vi "3667_Can_4Motor.vi"(0 "Device Number(Rl)":u8, 1 "Control Mode":T1, 2 "Rear Left Motor Inverted":bool, 3 "Rear Right Motor Inverted":bool, 5 "Device Number(Rr)":u8, 7 "Device Number(Fl)":u8, 9 "Device Number(Fr)":u8, 11 "error in (no error)":errorcluster, 13 "Front Left Motor Inverted":bool, 14 "Front Right Motor Inverted":bool) -> (4 "RobotDriveDevRef":T2={"DevStatus"={"status"=FALSE, "code"=0, "source"=""}, "Motors[]"=[], "Square Inputs"=FALSE, "Max Output"=1.0}, 15 "error out":errorcluster)   [LabVIEW 2016]
uses:
  <vilib>/Rock Robotics/WPI/RobotDrive/WPI_RobotDriveDevRef.ctl
  <vilib>/Rock Robotics/WPI/MotorControl/WPI_MotorControlDeviceRef.ctl
  <vilib>/Rock Robotics/WPI/MotorControl/WPI_MotorControlType.ctl
  <vilib>/Rock Robotics/SystemInterfaces/DIO/FPGA_DIOPWMChannel.ctl
  <vilib>/Rock Robotics/WPI/PWM/WPI_PWMDeadband.ctl
  <vilib>/Rock Robotics/WPI/ThirdParty/CanMotor/TalonSRX/WPI_CANTalonSRX_APIControlMode.ctl
  <vilib>/Rock Robotics/WPI/SafetyOutput/WPI_SafetyOutputConfigMenu.ctl
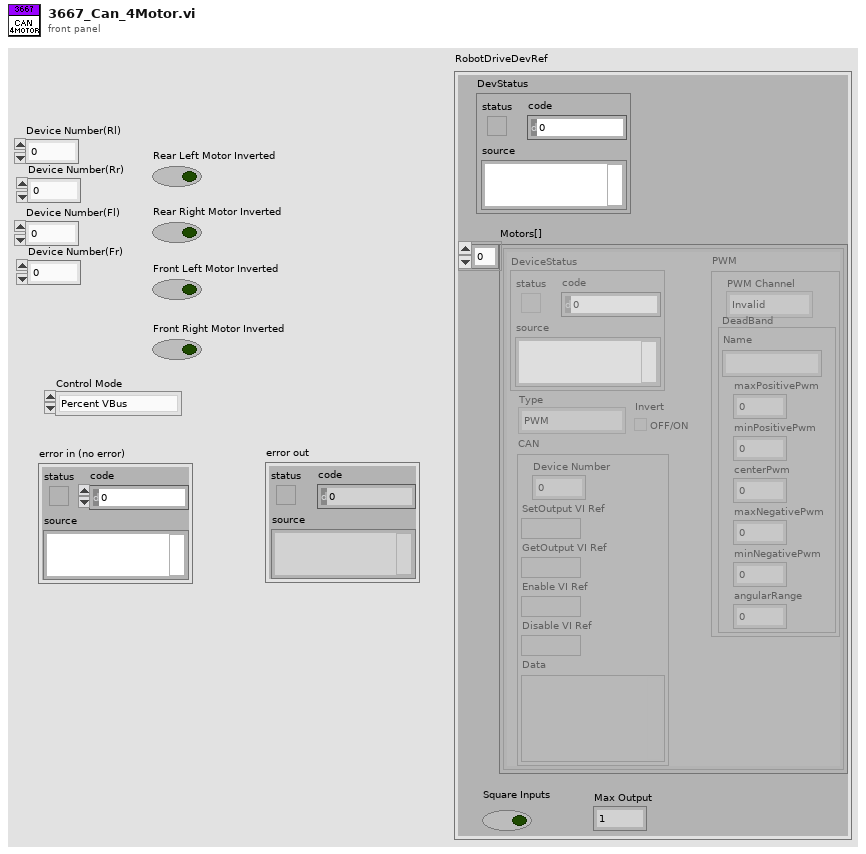
[diagram p1: front panel]
types:
  T1 = typedef "WPI_CANTalonSRX_APIControlMode.ctl" = enum8{"Percent VBus", "Speed", "Position", "Slave", "Unchanged / Invalid", "Voltage Compensation", "Current", "Motion Profile", "Motion Magic"}
  T2 = typedef "WPI_RobotDriveDevRef.ctl" = cluster{"DevStatus":errorcluster, "Motors[]":T3[], "Square Inputs":bool, "Max Output":dbl}
  T3 = typedef "WPI_MotorControlDeviceRef.ctl" = cluster{"DeviceStatus":errorcluster, "Type":T4, "PWM":cluster{"PWM Channel":T5, "DeadBand":T6}, "CAN":cluster{"Device Number":u8, "SetOutput VI Ref":variant, "GetOutput VI Ref":variant, "Enable VI Ref":variant, "Disable VI Ref":variant, "Data":variant}, "Invert":bool}
  T4 = typedef "WPI_MotorControlType.ctl" = enum16{"PWM", "CAN"}
  T5 = typedef "FPGA_DIOPWMChannel.ctl" = enum8{"PWM 0", "PWM 1", "PWM 2", "PWM 3", "PWM 4", "PWM 5", "PWM 6", "PWM 7", "PWM 8", "PWM 9", "PWM MXP 0", "PWM MXP 1", "PWM MXP 2", "PWM MXP 3", "PWM MXP 4", "PWM MXP 5", "PWM MXP 6", "PWM MXP 7", "PWM MXP 8", "PWM MXP 9", "Invalid"}
  T6 = typedef "WPI_PWMDeadband.ctl" = cluster{"Name":string, "maxPositivePwm":i32, "minPositivePwm":i32, "centerPwm":i32, "maxNegativePwm":i32, "minNegativePwm":i32, "angularRange":u16}
  T7 = typedef "WPI_SafetyOutputConfigMenu.ctl" = enum16{"Enable", "Disable"}
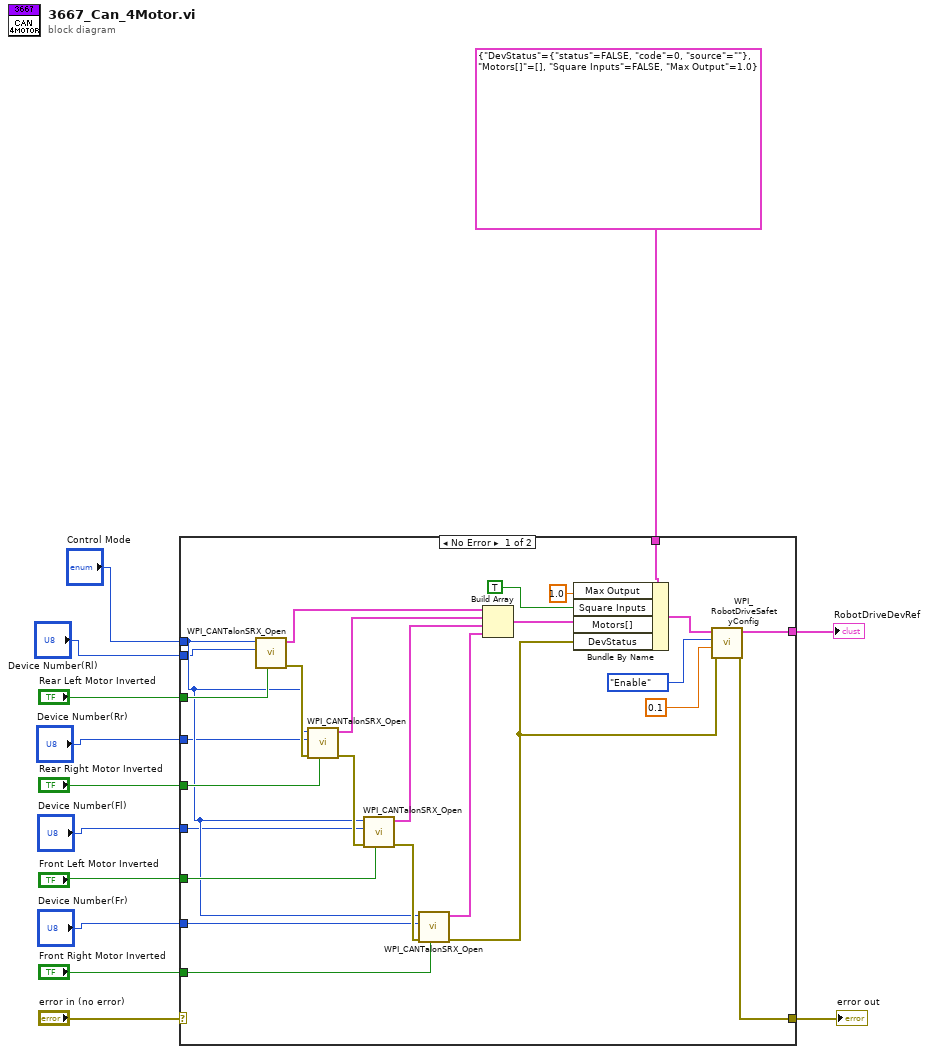
[diagram p0: block diagram]
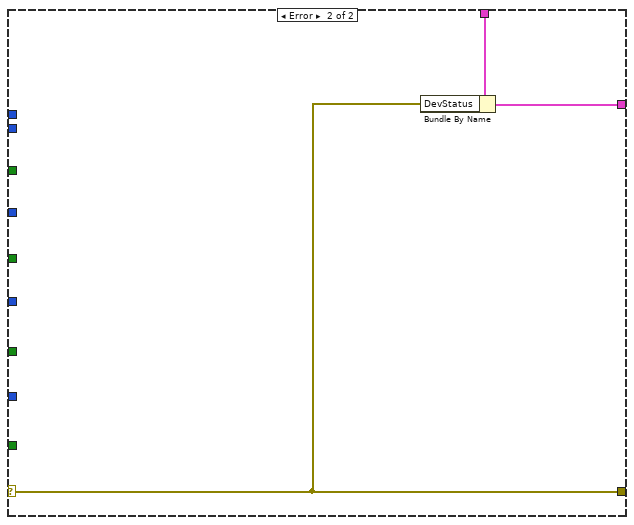
[diagram p2: hidden frame]
diagram:
  n1 = case shown="No Error" "error in (no error)" {
    selector: "error in (no error)" -> [_ w40]
    tunnel: [w21 w41] -> w13
    tunnel: T2 {"DevStatus"={"status"=FALSE, "code"=0, "source"=""}, "Motors[]"=[], "Square Inputs"=FALSE, "Max Output"=1.0} ("RobotDriveDevRef") -> [w39 w42]
    tunnel: "Rear Left Motor Inverted" -> [w29 _]
    tunnel: "Rear Right Motor Inverted" -> [w28 _]
    tunnel: "Front Right Motor Inverted" -> [w26 _]
    tunnel: "Front Left Motor Inverted" -> [w27 _]
    tunnel: [w22 w40] -> w6
    tunnel: "Control Mode" -> [w18 _]
    tunnel: "Device Number(Rl)" -> [w17 _]
    tunnel: "Device Number(Rr)" -> [w16 _]
    tunnel: "Device Number(Fl)" -> [w15 _]
    tunnel: "Device Number(Fr)" -> [w14 _]
    frame No Error {
      n2 = call <vilib>:"WPI_CANTalonSRX_Open.vi"("Invert"=w29, "Device Number"=w17, "Control Mode"=w18) -> ("error out"=w31:errorcluster, "CAN Talon SRX Ref"=w37:T3)  [unwired: 7 in]
      n3 = call <vilib>:"WPI_CANTalonSRX_Open.vi"("Invert"=w28, "error in"=w31, "Device Number"=w16, "Control Mode"=w18) -> ("error out"=w32:errorcluster, "CAN Talon SRX Ref"=w36:T3)  [unwired: 6 in]
      n4 = call <vilib>:"WPI_CANTalonSRX_Open.vi"("Invert"=w27, "error in"=w32, "Device Number"=w15, "Control Mode"=w18) -> ("error out"=w33:errorcluster, "CAN Talon SRX Ref"=w35:T3)  [unwired: 6 in]
      n5 = call <vilib>:"WPI_CANTalonSRX_Open.vi"("Invert"=w26, "error in"=w33, "Device Number"=w14, "Control Mode"=w18) -> ("error out"=w23:errorcluster, "CAN Talon SRX Ref"=w34:T3)  [unwired: 6 in]
      n6 = Build Array(w37, w36, w35, w34) -> (w30:T3[])
      n7 = Bundle By Name(cluster=w39, "Max Output"=1.0, "Square Inputs"=TRUE ("DestroyPWM?"), "Motors[]"=w30, "DevStatus"=w23) -> (w24:T2)
      n8 = call <vilib>:"WPI_RobotDriveSafetyConfig.vi"("error in (no error)"=w23, "timeout (s)"=0.1, "mode"=WPI_SafetyOutputConfigMenu."Enable", "RobotDriveDevRef"=w24) -> ("error out"=w22:errorcluster, "RobotDriveDevRef"=w21:T2)  [unwired: 6 out]
    }
    frame Error {
      n9 = Bundle By Name(cluster=w42, "DevStatus"=w40) -> (w41:T2)
    }
  }
  "RobotDriveDevRef" <- w13
  "error out" <- w6
